vi "FTW-JSON-Object-Update.vi"(0 "JSON Object":refnum<class "FTW-Container.lvclass">, 5 "JSON Object to Merge":string, 7 "Update Mode":T1, 11 "error in":errorcluster) -> (4 "JSON Object out":refnum<class "FTW-Container.lvclass">, 15 "error out":errorcluster)   [LabVIEW 2015]
uses:
  container/FTW-Container.lvclass
  FTW-JSON-JoinMode.ctl
panel:
  # "Inputs"
  # "Outputs"
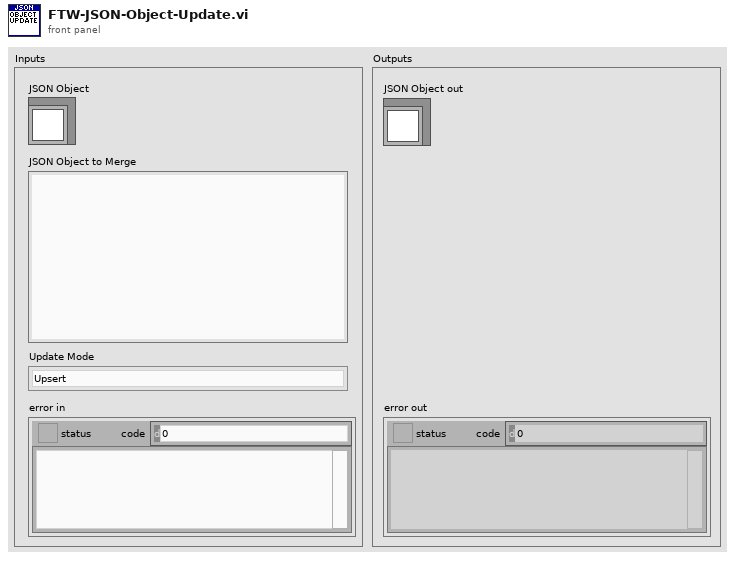
[diagram p1: front panel]
types:
  T1 = typedef "FTW-JSON-JoinMode.ctl" = enum32{"Upsert", "Update Only", "Insert Only"}
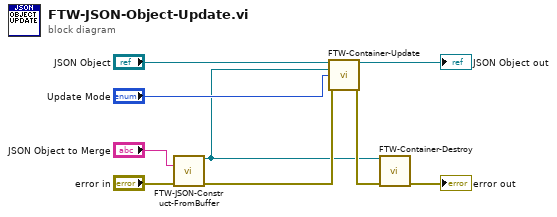
[diagram p0: block diagram]
diagram:
  n1 = call "FTW-JSON-Construct-FromBuffer.vi"("JSON String (UTF-8)"="JSON Object to Merge", "error in"="error in") -> ("JSON"=w1:refnum<class "FTW-Container.lvclass">, "error out"=w3:errorcluster)  [unwired: 12 in]
  n2 = call "FTW-Container-Update.vi"("FTW-Container In"="JSON Object", "Other Container"=w1, "Join Mode"="Update Mode", "error in"=w3) -> ("Updated Container"=→"JSON Object out":refnum<class "FTW-Container.lvclass">, "error out"=w2:errorcluster)  [unwired: 10 in]
  n3 = call "FTW-Container-Destroy.vi"("FTW-Container In"=w1, "error in"=w2) -> ("error out"=→"error out":errorcluster)  [unwired: 11 in, 2 out]
